vi "Method3.vi"(8 "error in (no error)":errorcluster, 11 "Class 2 in":refnum<class "Class 2.lvclass">) -> (0 "error out":errorcluster, 3 "Class 2 out":refnum<class "Class 2.lvclass">)   [LabVIEW 2023, in "Class 2.lvclass"]
uses:
  Class 2.lvclass
  Class 2.lvclass/Class 2.ctl
panel:
  in  "message":string="Method 3, Class 2"
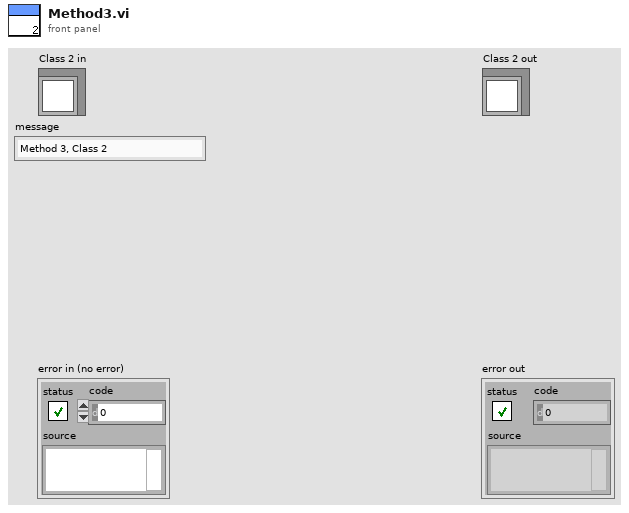
[diagram p1: front panel]
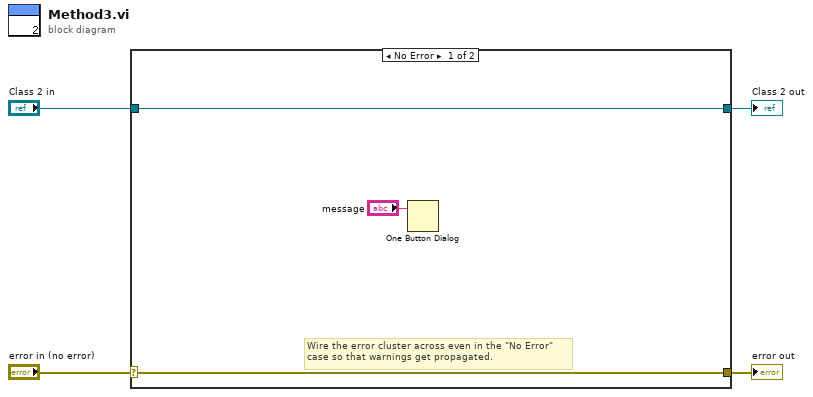
[diagram p0: block diagram]
diagram:
  n1 = case shown="No Error" "error in (no error)" {
    selector: "error in (no error)" -> [w6 w9]
    tunnel: [w6 w9] -> w3
    tunnel: [w7 w8] -> w1
    tunnel: "Class 2 in" -> [w7 w8]
    frame No Error {
      # "Wire the error cluster across even in the \"No Error\"\ncase so that warnings get propagated."
      n2 = One Button Dialog(message="message") -> ()  [unwired: 1 in, 1 out]
    }
    frame Error {
    }
  }
  "error out" <- w3
  "Class 2 out" <- w1
